vi "analog-transfer-test.vi"() -> ()   [LabVIEW 2019]
uses:
  <vilib>/Rock Robotics/WPI/ThirdParty/JAS_Junk/TrajLib/SlewRateLimiter_Execute.vi
  <vilib>/Rock Robotics/WPI/ThirdParty/JAS_Junk/TrajLib/SlewRateLimiter_New.vi
  <vilib>/Rock Robotics/WPI/ThirdParty/JAS_Junk/TrajLib/SlewRateLimiter_Reset.vi
  <vilib>/Rock Robotics/WPI/ThirdParty/JAS_Junk/TrajLib/SlewRateLimiter_Calculate.vi
  <vilib>/Rock Robotics/WPI/ThirdParty/JAS_Junk/TrajLib/SlewRateLimiter_SetRate.vi
  <vilib>/Rock Robotics/WPI/ThirdParty/JAS_Junk/TrajLib/Util_GetTime.vi
  <vilib>/Rock Robotics/WPI/ThirdParty/JAS_Junk/TrajLib/Trajectory_Library.lvlib
panel:
  in  "Tab Control":enum32{"Execution", "Logic"}(tab)
  out "Output":dbl
  in  "Rate 1":dbl=10.0
  in  "Input 1":dbl(slide)=10.0 scale=-100.0..100.0
  in  "Select":bool
  in  "Input 2":dbl(slide)=10.0 scale=-100.0..100.0
  in  "Rate 2":dbl=10.0
  out "Transfer":cluster{dbl, dbl, "Value_Output":dbl}(graph)
  # "Analog Value \nTransfer Test"
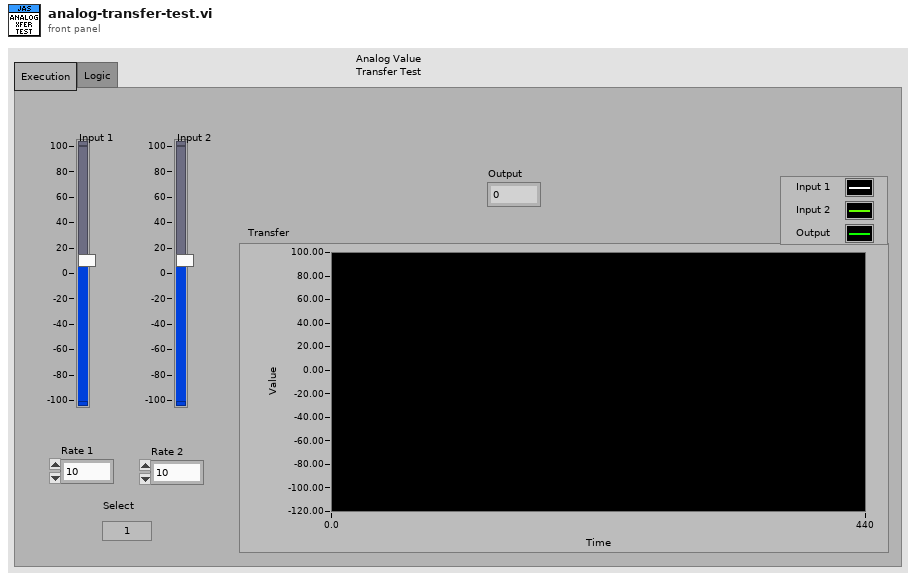
[diagram p1: front panel]
types:
  T1 = cluster{"Input 1":dbl, "Input 2":dbl, "Output":dbl}
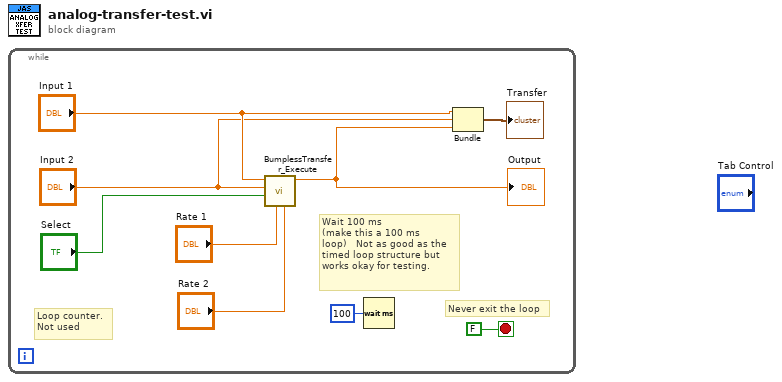
[diagram p0: block diagram]
diagram:
  n1 = while {
    stop <- FALSE stop-if-true
    # "Loop counter.\nNot used"
    # "Never exit the loop"
    # "Wait 100 ms\n(make this a 100 ms\nloop)   Not as good as the\ntimed loop structure but\nworks okay for testing."
    n2 = call <vilib>:"BumplessTransfer_Execute.vi"("Rate 2"="Rate 2", "Rate 1"="Rate 1", "Select 2"="Select", "Input 2"="Input 2", "Input 1"="Input 1") -> ("Output"=w2:dbl)  [unwired: 6 in]
    "Output" <- w2
    n3 = Wait (ms)(milliseconds to wait=u32 100) -> ()  [unwired: 1 out]
    n4 = Bundle("Input 1"="Input 1", "Input 2"="Input 2", "Output"=w2) -> (→"Transfer":T1)  [unwired: 1 in]
  }
